vi "Codepoint Array To String (Unicode).vi"(9 "error in":errorcluster, 10 "Codepoint Array":i32[](array[numeric]) format="%04x") -> (1 "error out":errorcluster, 2 "String":refnum<class "UTF-8 String.lvclass">)   [LabVIEW 2020, in "G-Unicode.lvlib"]
doc: "Converts an array of 32-bit integers representing Unicode codepoints into a UTF-8 String.\n\n<b>Codepoint Array</b> can also be a byte array of ASCII characters."
uses:
  G-Unicode.lvlib
  Types/UTF-8 String/UTF-8 String.lvclass
  Types/UTF-8 String/UTF-8 String.lvclass/UTF-8 String.ctl
  Private/Library/Result To Error.vi
  Private/Memory/Copy String.vi
  Private/Memory/Copy String.vi/4d47babd-4a2d-4eb7-b91b-7e707d692665.vi
  Private/Library/gu_free.vi
  <vilib>/Utility/error.llb/Error Cluster From Error Code.vi
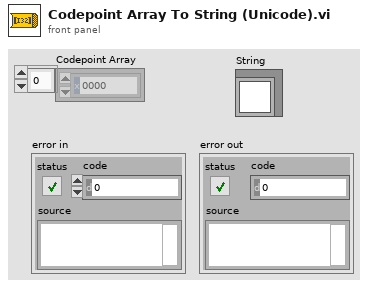
[diagram p1: front panel]
types:
  T1 = typedef "G-Unicode.lvlib/Encoded UTF-8 String.ctl" = string
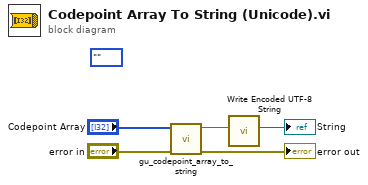
[diagram p0: block diagram]
diagram:
  (unwired) enum16{""}.""
  n1 = call "gu_codepoint_array_to_string.vi"("error in"="error in", "Codepoint Array"="Codepoint Array") -> ("error out"=→"error out":errorcluster, "Encoded String"=w4:T1)  [unwired: 8 in]
  n2 = call "Write Encoded UTF-8 String.vi"("Encoded UTF-8 String"=w4) -> ("UTF-8 String"=→"String":refnum<class "UTF-8 String.lvclass">)  [unwired: 10 in]
